vi "Hysteresis_min-LAPTOP-A1ILEVN9.vi"(0 "input":dbl, 2 "type":enum16{"percentage", "level"}(ring), 5 "Min":dbl=26.0 format="%#_13g", 7 "H":dbl=22.0 format="%#_13g", 11 "error in":errorcluster) -> (8 "Deviation":bool, 15 "error out":errorcluster)   [LabVIEW 2022 SP3]
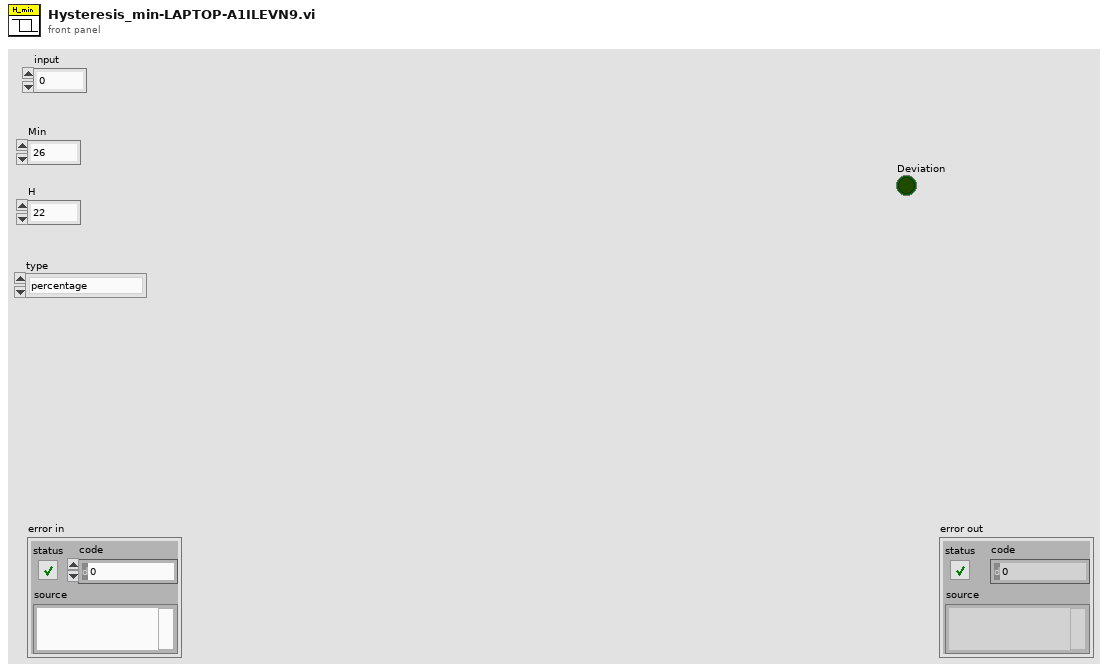
[diagram p1: front panel]
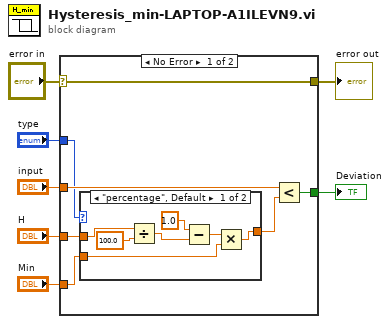
[diagram p0: block diagram]
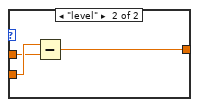
[diagram p2: hidden frame]
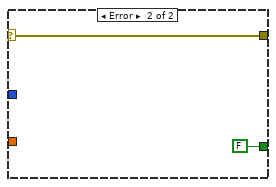
[diagram p3: hidden frame]
diagram:
  n1 = case shown="No Error" "error in" {
    selector: "error in" -> [w13 w26]
    tunnel: "H" -> [w9 _]
    tunnel: "input" -> [w14 _]
    tunnel: "Min" -> [w10 _]
    tunnel: [w13 w26] -> w3
    tunnel: [w12 FALSE] -> w2
    tunnel: "type" -> [w11 _]
    frame No Error {
      n2 = case shown="\"percentage\", Default" w11 {
        tunnel: w10 -> [w18 w24]
        tunnel: w9 -> [w16 w23]
        tunnel: [w15 w22] -> w8
        frame "percentage", Default {
          n3 = Divide(x=w16, y=100.0) -> (x/y=w20:dbl)
          n4 = Subtract(x=1.0 ("y"), y=w20) -> (x-y=w21:dbl)
          n5 = Multiply(x=w21, y=w18) -> (x*y=w15:dbl)
        }
        frame "level" {
          n6 = Subtract(x=w24, y=w23) -> (x-y=w22:dbl)
        }
      }
      n7 = Less?(x=w14, y=w8) -> (x < y?=w12:bool)
    }
    frame Error {
    }
  }
  "error out" <- w3
  "Deviation" <- w2
